vi "Test Arm Config.vi"() -> ()   [LabVIEW 2018]
uses:
  Arm Positions.ctl
  <vilib>/Utility/config.llb/Read Key (String).vi
  Implementation/Arm Published Globals.vi
  <vilib>/Utility/config.llb/NI_LVConfig.lvlib
  <vilib>/Utility/config.llb/Write Key (String).vi
panel:
  in  "Arm Positions":T1=enum."Hatch - High 2"
  in  "Read FIle":bool
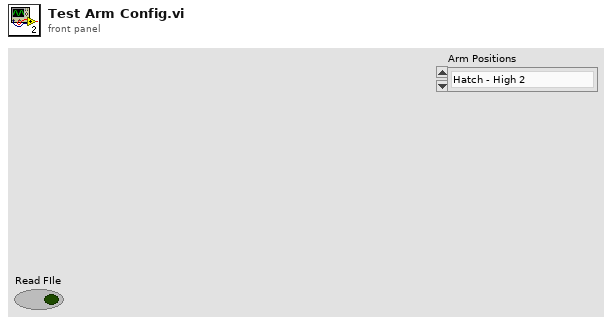
[diagram p1: front panel]
types:
  T1 = typedef "Arm Positions.ctl" = enum16{"Home Position", "Safe Position", "Hatch - Ground", "Hatch - Low", "Hatch - Middle", "Hatch - High", "Hatch - High 2", "Cargo - Low", "Cargo - Middle", "Cargo - High", "Cargo - Loading Station", "Hatch - Loading Station", "Cargo - Ground", "Turret - Left", "Turret - Front", "Turret - Right", "Turret - Back", "Climbing - Forward"}
  T2 = typedef "NI_LVConfig.lvlib/Config Data RefNum.ctl" = refnum<k1>
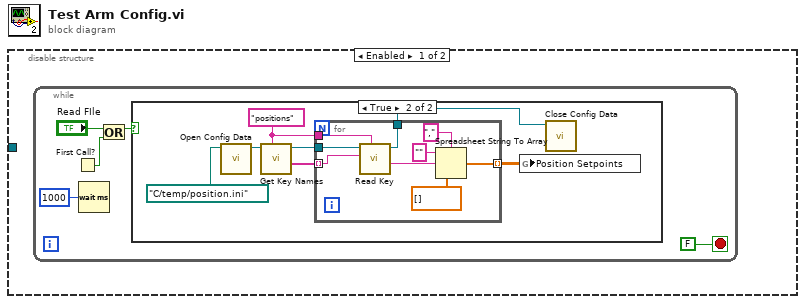
[diagram p0: block diagram]
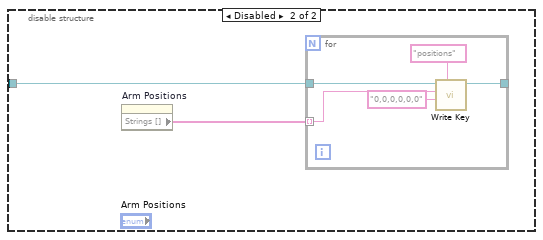
[diagram p3: hidden frame]
diagram:
  n1 = disable-structure shown="Enabled" {
    disable-tunnel: _ -> [_ w24]
    frame Enabled {
      n2 = while {
        stop <- FALSE stop-if-true
        n3 = First Call?() -> (First Call?: T/F=w2:bool)
        n4 = Wait (ms)(milliseconds to wait=u32 1000) -> ()  [unwired: 1 out]
        n5 = Or(x="Read FIle", y=w2) -> (x .or. y?=w3:bool)
        n6 = case shown="True" w3 {
          frame False {
          }
          frame True {
            w10 = "positions" ("section")
            n7 = call <vilib>:"Open Config Data.vi"("configuration file path"=path "C:/temp/position.ini") -> ("refnum"=w7:T2)  [unwired: 8 in, 2 out]
            n8 = call <vilib>:"Get Key Names.vi"("section"=w10, "refnum"=w7) -> ("key names"=w9:string[], "refnum out"=w12:T2)  [unwired: 6 in, 2 out]
            n9 = for {
              tunnel: w12 -> [w21]
              tunnel: [w18] -> w11 mode=indexing
              tunnel: w10 -> [w15]
              tunnel: w9 -> [w14] mode=indexing
              tunnel: [w13] -> w6
              n10 = call-poly <vilib>:"Read Key.vi"("section"=w15, "key"=w14, "refnum"=w21) -> ("value"=w19:string, "refnum out"=w13:T2)  [unwired: 5 in, 2 out]
              n11 = Spreadsheet String To Array(delimiter (Tab)=",", format string="", spreadsheet string=w19, array type (2D Dbl)=dbl[] []) -> (array=w18:dbl[])
            }
            n12 = global write "Arm Published Globals.vi" "Position Setpoints"(w11) -> ()
            n13 = call <vilib>:"Close Config Data.vi"("refnum"=w6) -> ()  [unwired: 9 in, 2 out]
          }
        }
      }
    }
    frame Disabled {
      n14 = property on="Arm Positions" class="Enum (strict)"() -> ("Strings []"=w23:string[])  [unwired: 2 in, 2 out]
      n15 = for {
        tunnel: w24 -> [w29]
        tunnel: w23 -> [w27] mode=indexing
        tunnel: [w25] -> w22
        n16 = call-poly <vilib>:"Write Key.vi"("section"="positions", "value"="0,0,0,0,0,0", "key"=w27, "refnum"=w29) -> ("refnum out"=w25:T2)  [unwired: 5 in, 2 out]
      }
    }
  }
